vi "Assign COM Port to Aircraft.vi"(8 "error out":errorcluster, 11 "Aircraft COM Port":refnum<visa-resource-name>) -> (0 "error out 2":errorcluster, 1 "Aircraft ID":u8, 2 "Message Complete":bool, 3 "Aircraft COM Port 2":refnum<visa-resource-name>)   [LabVIEW 2014]
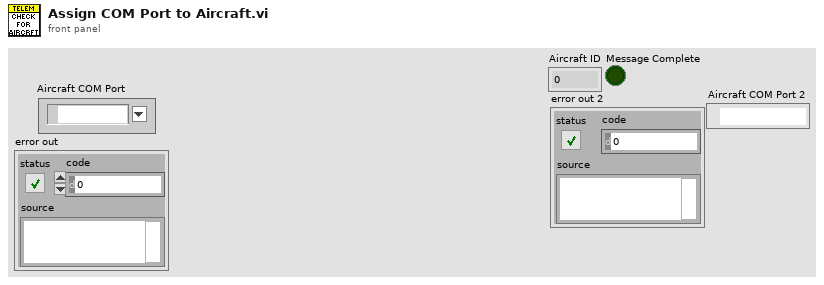
[diagram p1: front panel]
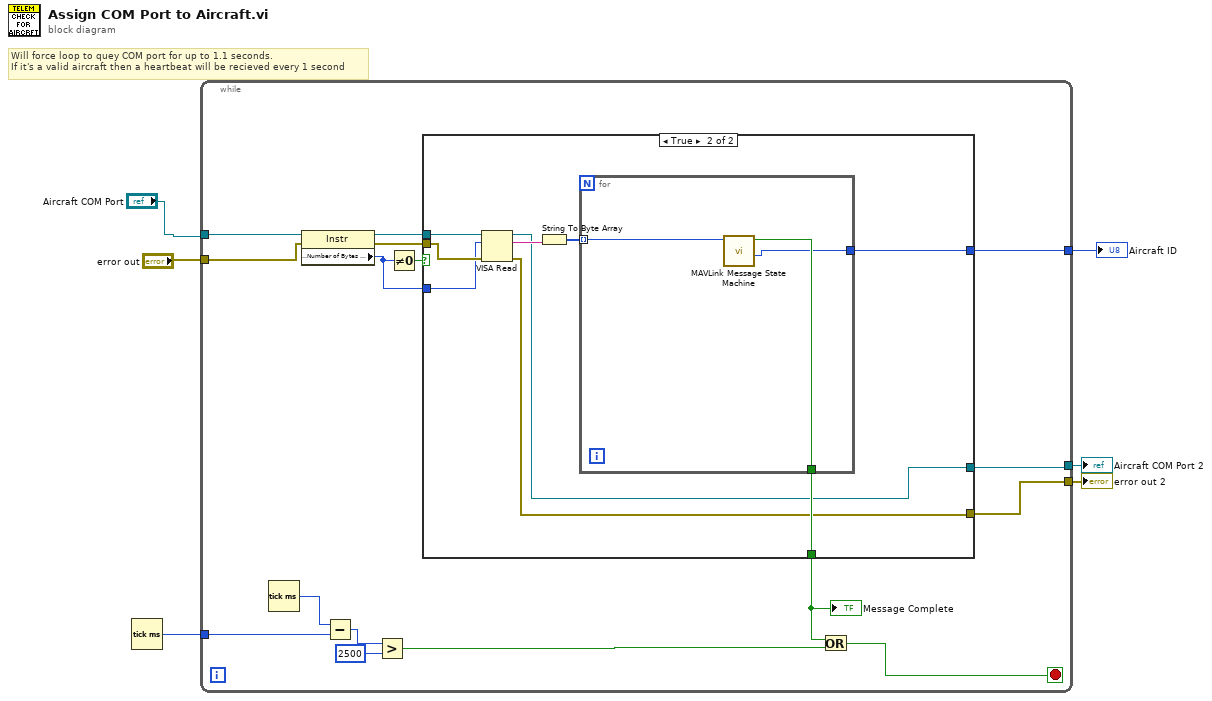
[diagram p0: block diagram]
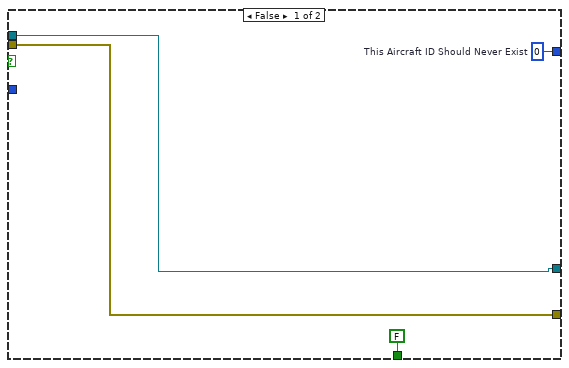
[diagram p2: hidden frame]
diagram:
  # "Will force loop to quey COM port for up to 1.1 seconds.\nIf it's a valid aircraft then a heartbeat will be recieved every 1 second"
  n1 = Tick Count (ms)() -> (millisecond timer value=w1:u32)
  n2 = while {
    tunnel: "Aircraft COM Port" -> [w22]
    tunnel: "error out" -> [w21]
    tunnel: [w16] -> w4
    tunnel: [w15] -> w3
    tunnel: [w14] -> w2
    tunnel: w1 -> [w10]
    stop <- w12 stop-if-true
    n3 = Tick Count (ms)() -> (millisecond timer value=w11:u32)
    n4 = property class="Instr"(reference=w22, error in=w21) -> (reference out=w19:refnum<visa-resource-name>, error out=w18:errorcluster, "Serial Settings:Number of Bytes at Serial Port"=w17:u32)
    n5 = Subtract(x=w11, y=w10) -> (x-y=w9:u32)
    n6 = Greater?(x=w9, y=u32 2500) -> (0:w7:bool)
    n7 = Not Equal To 0?(x=w17) -> (x != 0?=w20:bool)
    n8 = case shown="True" w20 {
      tunnel: w19 -> [w23 w35]
      tunnel: w18 -> [w24 w34]
      tunnel: w17 -> [_ w33]
      tunnel: [FALSE ("Message Complete") w30] -> w13
      tunnel: [w25 w29] -> w16
      tunnel: [w24 w28] -> w15
      tunnel: [w23 w27] -> w14
      frame False {
        w25 = u8 0  # This Aircraft ID Should Never Exist
      }
      frame True {
        n9 = VISA Read(VISA resource name=w35, byte count=w33, error in (no error)=w34) -> (VISA resource name out=w27:refnum<visa-resource-name>, read buffer=w32:string, error out=w28:errorcluster)  [unwired: 1 out]
        n10 = String To Byte Array(string=w32) -> (unsigned byte array=w31:u8[])
        n11 = for {
          tunnel: w31 -> [w38] mode=indexing
          tunnel: [w37] -> w30
          tunnel: [w36] -> w29
          n12 = call "MAVLink Message State Machine.vi"("Incoming Bytes"=w38) -> ("Aircraft ID"=w36:u8, "Message Complete"=w37:bool)  [unwired: 7 in, 2 out]
        }
      }
    }
    "Message Complete" <- w13
    n13 = Or(x=w13, y=w7) -> (x .or. y?=w12:bool)
  }
  "Aircraft ID" <- w4
  "error out 2" <- w3
  "Aircraft COM Port 2" <- w2
